vi "Read File.vi"(8 "error in (no error)":errorcluster, 10 "Path in":path, 11 "Reflective Memory File in":refnum<class "Reflective Memory File.lvclass">) -> (0 "error out":errorcluster, 2 "SysDef":T1 {"Tree"."Properties"."Type" items=["K_STRING", "K_BOOL", "K_I32", "K_U32", "K_DOUBLE", "K_U64", "K_VARIANT", "K_DEPENDENTFILE", "K_DEPENDENTNODE", "K_DATASOURCENODE", "K_U16", "K_DBLARR", "K_U32ARR", "K_I32ARR", "K_STRINGARR", "K_DICTIONARY", "K_DICTIONARYARR"]})   [LabVIEW 2015, in "RefMem DMA Custom Device.lvlib" / "Reflective Memory File.lvclass"]
uses:
  Reflective Memory File.lvclass
  <vilib>/NI/NI VeriStand Advanced SysDef API/_Types/SysDef.Export.ctl
  <vilib>/NI/NI VeriStand Advanced SysDef API/_Types/TreeItem.ctl
  <vilib>/NI/NI VeriStand Advanced SysDef API/_Types/TreeItem.Info.ctl
  <vilib>/NI Veristand/Custom Device API/Custom Device Channel.ctl
  <vilib>/NI Veristand/Custom Device API/Custom Device Channel Type.ctl
  <vilib>/NI Veristand/Custom Device API/Custom Device Waveform.ctl
  <vilib>/NI Veristand/Custom Device API/Custom Device Waveform DataType.ctl
  <vilib>/NI/NI VeriStand Advanced SysDef API/_Types/TreeItem.Property.ctl
  <vilib>/Utility/file.llb/Read Delimited Spreadsheet (string).vi
  Controls/Global.vi
  <vilib>/NI Veristand/Custom Device API/Custom Device API.lvlib
  <vilib>/NI/NI VeriStand Advanced SysDef API/SysDef API/Advanced System Definition.lvlib
  RefMem DMA Custom Device.lvlib
panel:
  out "deleted portion":string[](array[string])
  out "array w/ subset deleted":string[][](array[string])
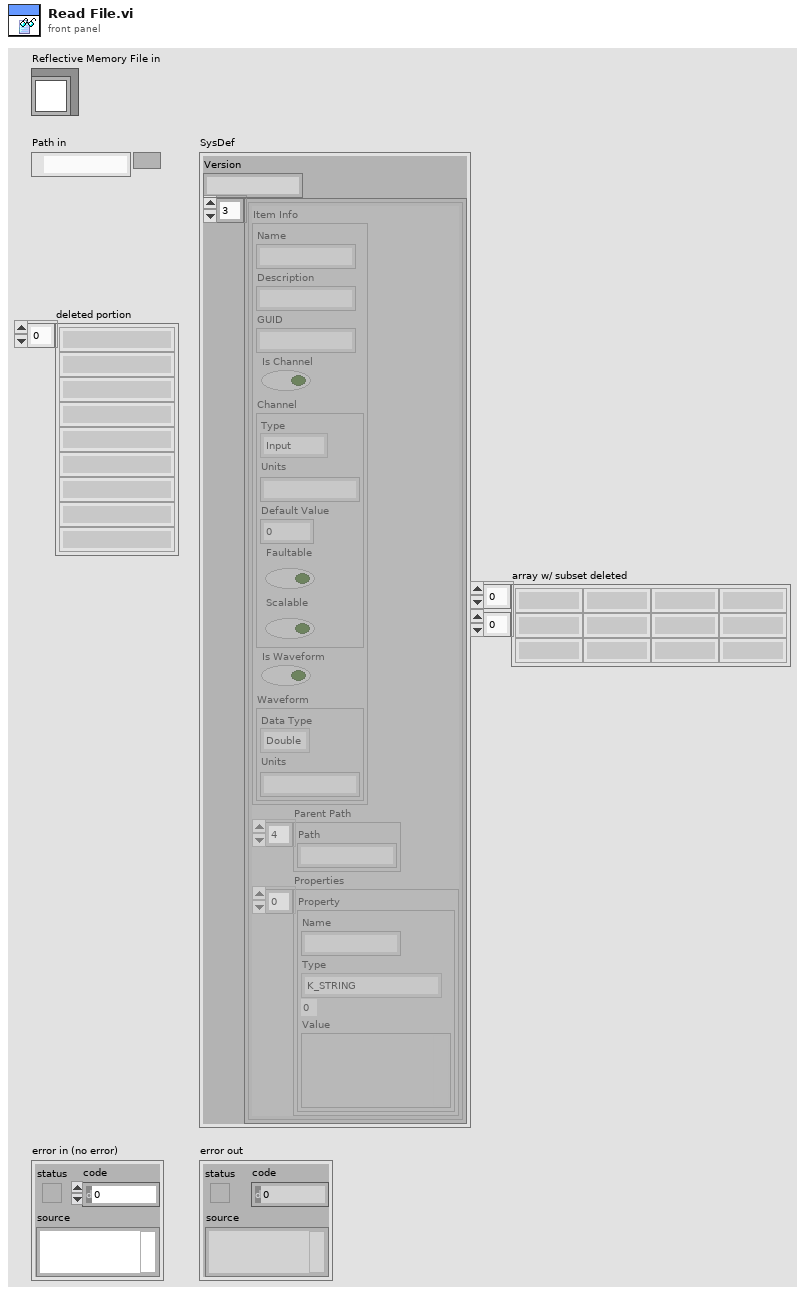
[diagram p1: front panel]
types:
  T1 = typedef "Advanced System Definition.lvlib/SysDef.Export.ctl" = cluster{"Version":string, "Tree":T2[]}
  T2 = typedef "Advanced System Definition.lvlib/TreeItem.ctl" = cluster{"Item Info":T3, "Parent Path":string[], "Properties":T8[]}
  T3 = typedef "Advanced System Definition.lvlib/TreeItem.Info.ctl" = cluster{"Name":string, "Description":string, "GUID":string, "Is Channel":bool, "Channel":T4, "Is Waveform":bool, "Waveform":T6}
  T4 = typedef "Custom Device API.lvlib/Custom Device Channel.ctl" = cluster{"Type":T5, "Units":string, "Default Value":dbl, "Faultable":bool, "Scalable":bool}
  T5 = typedef "Custom Device API.lvlib/Custom Device Channel Type.ctl" = enum16{"Input", "Output"}
  T6 = typedef "Custom Device API.lvlib/Custom Device Waveform.ctl" = cluster{"Data Type":T7, "Units":string}
  T7 = typedef "Custom Device API.lvlib/Custom Device Waveform DataType.ctl" = enum16{"Double", "Complex Double"}
  T8 = typedef "Advanced System Definition.lvlib/TreeItem.Property.ctl" = cluster{"Name":string, "Type":i32, "Value":variant}
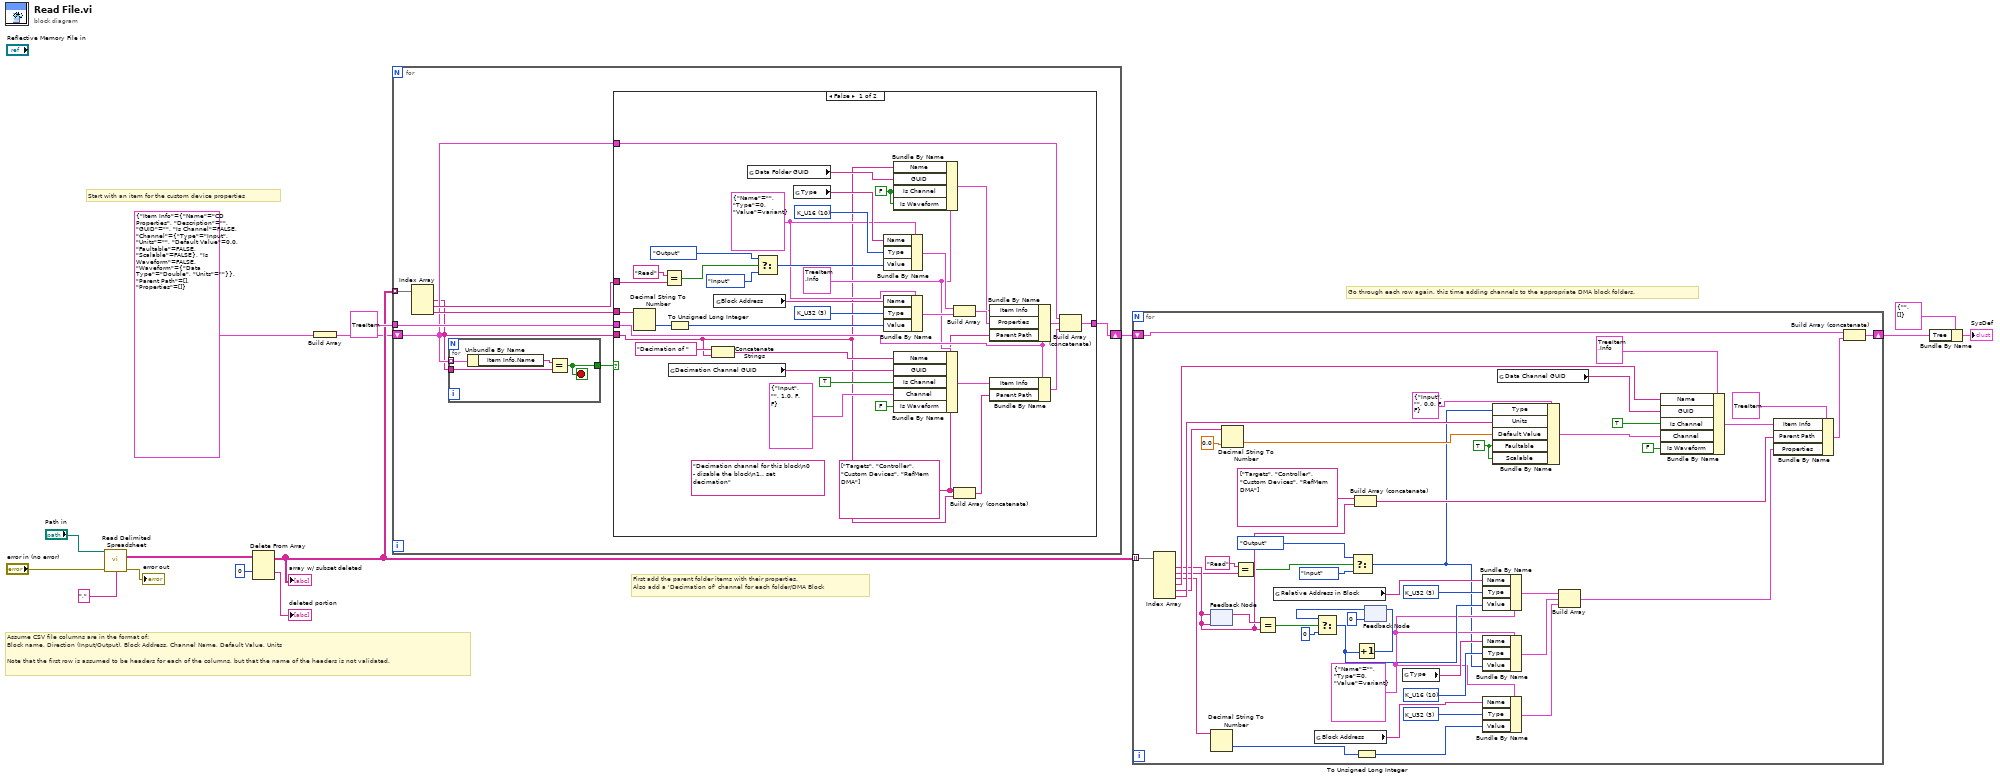
[diagram p0: block diagram]
diagram:
  # "Go through each row again, this time adding channels to the appropriate DMA block folders."
  # "First add the parent folder items with their properties.\nAlso add a 'Decimation of' channel for each folder/DMA Block"
  # "Assume CSV file columns are in the format of:\nBlock name, Direction (Input/Output), Block Address, Channel Name, Default Value, Units\n\nNote that the first row is assumed to be headers for each of the columns, but that the name of the headers is not validated."
  # "Start with an item for the custom device properties"
  n1 = call-poly <vilib>:"Read Delimited Spreadsheet.vi"("file path (dialog if empty)"="Path in", "error in (no error)"="error in (no error)", "delimiter (\\t)"="," ("delimiter (\\t)")) -> ("all rows"=w14:string[][], "error out"=→"error out":errorcluster)  [unwired: 7 in, 4 out]
  n2 = Delete From Array(array=w14, index (row)=0) -> (deleted portion=→"deleted portion":string[], array with subset deleted=w5:string[][])  [unwired: 2 in]
  "array w/ subset deleted" <- w5
  n3 = Build Array(T2 {"Item Info"={"Name"="CD Properties", "Description"="", "GUID"="", "Is Channel"=FALSE, "Channel"={"Type"=enum."Input", "Units"="", "Default Value"=0.0, "Faultable"=FALSE, "Scalable"=FALSE}, "Is Waveform"=FALSE, "Waveform"={"Data Type"=enum."Double", "Units"=""}}, "Parent Path"=[], "Properties"=[]} ("TreeItem")) -> (w1:T2[])
  n4 = for {
    tunnel: w5 -> [w22] mode=indexing
    shift-right: [w20] -> w6
    shift-left: w1 -> [w18]
    tunnel: T2 {"Item Info"={"Name"="", "Description"="", "GUID"="", "Is Channel"=FALSE, "Channel"={"Type"=enum."Input", "Units"="", "Default Value"=0.0, "Faultable"=FALSE, "Scalable"=FALSE}, "Is Waveform"=FALSE, "Waveform"={"Data Type"=enum."Double", "Units"=""}}, "Parent Path"=[], "Properties"=[]} ("TreeItem") -> [w23]
    n5 = Index Array(array=w22) -> (element #1=w17:string, element #2=w21:string, element #3=w19:string)  [unwired: 3 in]
    n6 = for {
      tunnel: w18 -> [w64] mode=indexing
      tunnel: w17 -> [w62]
      tunnel: [w61] -> w16
      stop <- w61 stop-if-true
      n7 = Unbundle By Name(w64) -> ("Item Info.Name"=w63:string)
      n8 = Equal?(x=w63, y=w62) -> (x = y?=w61:bool)
    }
    n9 = case shown="False" w16 {
      tunnel: w23 -> [w32 _]
      tunnel: w21 -> [w55 _]
      tunnel: [w45 w60] -> w20
      tunnel: w19 -> [w44 _]
      tunnel: w18 -> [w37 w60]
      tunnel: w17 -> [w26 _]
      frame False {
        w24 = string[] ["Targets", "Controller", "Custom Devices", "RefMem DMA"]
        (unwired) "Decimation channel for this block\n0 - disable the block\n1.. set decimation" ("Section Name")
        w40 = 3 items=["K_STRING", "K_BOOL", "K_I32", "K_U32", "K_DOUBLE", "K_U64", "K_VARIANT", "K_DEPENDENTFILE", "K_DEPENDENTNODE", "K_DATASOURCENODE", "K_U16", "K_DBLARR", "K_U32ARR", "K_I32ARR", "K_STRINGARR", "K_DICTIONARY", "K_DICTIONARYARR"] ("Type")
        w56 = 10 items=["K_STRING", "K_BOOL", "K_I32", "K_U32", "K_DOUBLE", "K_U64", "K_VARIANT", "K_DEPENDENTFILE", "K_DEPENDENTNODE", "K_DATASOURCENODE", "K_U16", "K_DBLARR", "K_U32ARR", "K_I32ARR", "K_STRINGARR", "K_DICTIONARY", "K_DICTIONARYARR"] ("Type")
        w43 = T8 {"Name"="", "Type"=0, "Value"=variant} ("Property")
        w59 = FALSE ("Is Channel")
        w30 = T3 {"Name"="", "Description"="", "GUID"="", "Is Channel"=FALSE, "Channel"={"Type"=enum."Input", "Units"="", "Default Value"=0.0, "Faultable"=FALSE, "Scalable"=FALSE}, "Is Waveform"=FALSE, "Waveform"={"Data Type"=enum."Double", "Units"=""}} ("Item Info")
        n10 = Decimal String To Number(string=w44) -> (number=w39:i32)  [unwired: 2 in, 1 out]
        n11 = Equal?(x="Read", y=w55) -> (x = y?=w53:bool)
        n12 = global read "Global.vi" "Decimation Channel GUID"() -> (w34:string)
        n13 = To Unsigned Long Integer(number=w39) -> (unsigned 32bit integer=w38:u32)
        n14 = Concatenate Strings("Decimation of " ("string"), w26) -> (w35:string)
        n15 = global read "Global.vi" "Block Address"() -> (w41:string)
        n16 = global read "Global.vi" "Data Folder GUID"() -> (w58:string)
        n17 = Select(t=Custom_Device_Channel_Type."Output" ("Type"), s=w53, f=Custom_Device_Channel_Type."Input" ("Type")) -> (s? t:f=w50:T5)
        n18 = global read "Global.vi" "Type"() -> (w57:string)
        n19 = Bundle By Name(cluster=w43, "Name"=w57, "Type"=w56, "Value"=w50) -> (w49:T8)
        n20 = Bundle By Name(cluster=w43, "Name"=w41, "Type"=w40, "Value"=w38) -> (w42:T8)
        n21 = Bundle By Name(cluster=w30, "Name"=w26, "GUID"=w58, "Is Channel"=w59, "Is Waveform"=w59) -> (w47:T3)
        n22 = Bundle By Name(cluster=w30, "Name"=w35, "GUID"=w34, "Is Channel"=TRUE, "Channel"=T4 {"Type"=enum."Input", "Units"="", "Default Value"=1.0, "Faultable"=FALSE, "Scalable"=FALSE}, "Is Waveform"=FALSE) -> (w31:T3)
        n23 = Build Array(w49, w42) -> (w48:T8[])
        n24 = Build Array (concatenate)(w24, w26) -> (w25:string[])
        n25 = Bundle By Name(cluster=w32, "Item Info"=w47, "Properties"=w48, "Parent Path"=w24) -> (w46:T2)
        n26 = Bundle By Name(cluster=w32, "Item Info"=w31, "Parent Path"=w25) -> (w29:T2)
        n27 = Build Array (concatenate)(w37, w46, w29) -> (w45:T2[])
      }
      frame True {
      }
    }
  }
  n28 = for {
    tunnel: w5 -> [w111] mode=indexing
    shift-right: [w70] -> w4
    shift-left: w6 -> [w69]
    w82 = 10 items=["K_STRING", "K_BOOL", "K_I32", "K_U32", "K_DOUBLE", "K_U64", "K_VARIANT", "K_DEPENDENTFILE", "K_DEPENDENTNODE", "K_DATASOURCENODE", "K_U16", "K_DBLARR", "K_U32ARR", "K_I32ARR", "K_STRINGARR", "K_DICTIONARY", "K_DICTIONARYARR"] ("Type")
    w78 = 3 items=["K_STRING", "K_BOOL", "K_I32", "K_U32", "K_DOUBLE", "K_U64", "K_VARIANT", "K_DEPENDENTFILE", "K_DEPENDENTNODE", "K_DATASOURCENODE", "K_U16", "K_DBLARR", "K_U32ARR", "K_I32ARR", "K_STRINGARR", "K_DICTIONARY", "K_DICTIONARYARR"] ("Type")
    w90 = 3 items=["K_STRING", "K_BOOL", "K_I32", "K_U32", "K_DOUBLE", "K_U64", "K_VARIANT", "K_DEPENDENTFILE", "K_DEPENDENTNODE", "K_DATASOURCENODE", "K_U16", "K_DBLARR", "K_U32ARR", "K_I32ARR", "K_STRINGARR", "K_DICTIONARY", "K_DICTIONARYARR"] ("Type")
    w76 = T8 {"Name"="", "Type"=0, "Value"=variant} ("Property")
    w105 = TRUE ("Faultable")
    n29 = Index Array(array=w111) -> (element #1=w95:string, element #2=w83:string, element #3=w80:string, element #4=w110:string, element #5=w102:string, element #6=w104:string)  [unwired: 6 in]
    n30 = feedback-in #1(w95) -> ()
    n31 = feedback #1(w95) -> (w96:string)
    n32 = Decimal String To Number(string=w80) -> (number=w81:i32)  [unwired: 2 in, 1 out]
    n33 = Decimal String To Number(string=w102, default (0L)=0.0) -> (number=w101:dbl)  [unwired: 1 in, 1 out]
    n34 = Equal?(x="Read", y=w83) -> (x = y?=w85:bool)
    n35 = Equal?(x=w96, y=w95) -> (x = y?=w94:bool)
    n36 = global read "Global.vi" "Relative Address in Block"() -> (w91:string)
    n37 = global read "Global.vi" "Block Address"() -> (w77:string)
    n38 = Select(t=Custom_Device_Channel_Type."Output" ("Type"), s=w85, f=Custom_Device_Channel_Type."Input" ("Type")) -> (s? t:f=w68:T5)
    n39 = Build Array (concatenate)(string[] ["Targets", "Controller", "Custom Devices", "RefMem DMA"], w95) -> (w97:string[])
    n40 = To Unsigned Long Integer(number=w81) -> (unsigned 32bit integer=w79:u32)
    n41 = feedback #2(u32 0) -> (w67:u32)
    n42 = Select(t=w67, s=w94, f=u32 0 ("t")) -> (s? t:f=w89:u32)
    n43 = Increment(x=w89) -> (x+1=w92:u32)
    n44 = feedback-in #2(w92) -> ()
    n45 = global read "Global.vi" "Type"() -> (w88:string)
    n46 = Bundle By Name(cluster=w76, "Name"=w91, "Type"=w90, "Value"=w89) -> (w75:T8)
    n47 = Bundle By Name(cluster=w76, "Name"=w88, "Type"=w82, "Value"=w68) -> (w74:T8)
    n48 = Bundle By Name(cluster=w76, "Name"=w77, "Type"=w78, "Value"=w79) -> (w73:T8)
    n49 = Bundle By Name(cluster=T4 {"Type"=enum."Input", "Units"="", "Default Value"=0.0, "Faultable"=FALSE, "Scalable"=FALSE} ("Channel"), "Type"=w68, "Units"=w104, "Default Value"=w101, "Faultable"=w105, "Scalable"=w105) -> (w100:T4)
    n50 = global read "Global.vi" "Data Channel GUID"() -> (w109:string)
    n51 = Build Array(w75, w74, w73) -> (w72:T8[])
    n52 = Bundle By Name(cluster=T3 {"Name"="", "Description"="", "GUID"="", "Is Channel"=FALSE, "Channel"={"Type"=enum."Input", "Units"="", "Default Value"=0.0, "Faultable"=FALSE, "Scalable"=FALSE}, "Is Waveform"=FALSE, "Waveform"={"Data Type"=enum."Double", "Units"=""}} ("Item Info"), "Name"=w110, "GUID"=w109, "Is Channel"=TRUE, "Channel"=w100, "Is Waveform"=FALSE) -> (w98:T3)
    n53 = Bundle By Name(cluster=T2 {"Item Info"={"Name"="", "Description"="", "GUID"="", "Is Channel"=FALSE, "Channel"={"Type"=enum."Input", "Units"="", "Default Value"=0.0, "Faultable"=FALSE, "Scalable"=FALSE}, "Is Waveform"=FALSE, "Waveform"={"Data Type"=enum."Double", "Units"=""}}, "Parent Path"=[], "Properties"=[]} ("TreeItem"), "Item Info"=w98, "Parent Path"=w97, "Properties"=w72) -> (w71:T2)
    n54 = Build Array (concatenate)(w69, w71) -> (w70:T2[])
  }
  n55 = Bundle By Name(cluster=T1 {"Version"="", "Tree"=[]} ("SysDef"), "Tree"=w4) -> (→"SysDef":T1)
